vi "Camera Params OFF_Luan2024.05.01.vi"(8 "error in (no error)":errorcluster, 11 "IMAQDx session In":T1) -> (0 "error out":errorcluster, 3 "IMAQDx session out":T1)   [LabVIEW 2023]
uses:
  <vilib>/userDefined/High Color/IMAQdx.ctl
  <resource>/objmgr/imaqdx.rc
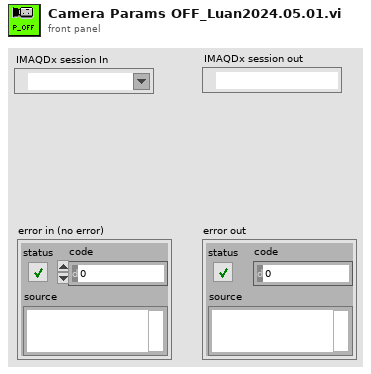
[diagram p1: front panel]
types:
  T1 = typedef "IMAQdx.ctl" = refnum<k21>
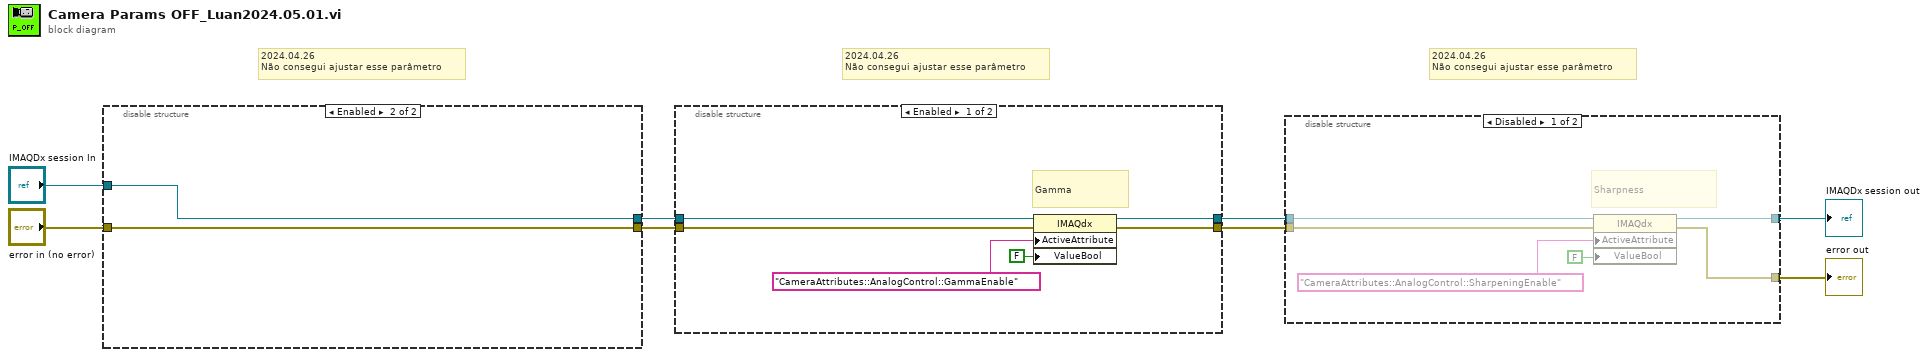
[diagram p0: block diagram]
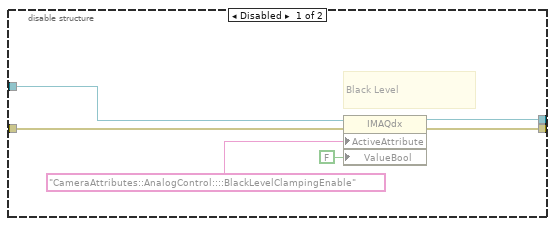
[diagram p4: hidden frame]
diagram:
  # "2024.04.26\nNão consegui ajustar esse parâmetro"
  # "2024.04.26\nNão consegui ajustar esse parâmetro"
  # "2024.04.26\nNão consegui ajustar esse parâmetro"
  n1 = disable-structure shown="Enabled" {
    disable-tunnel: [w14 w15] -> w6
    disable-tunnel: [w13 w16] -> w5
    disable-tunnel: "IMAQDx session In" -> [w11 w16]
    disable-tunnel: "error in (no error)" -> [w10 w15]
    frame Disabled {
      # "Black Level"
      n2 = property class="IMAQdx"(reference=w11, error in=w10, "ActiveAttribute"="CameraAttributes::AnalogControl::::BlackLevelClampingEnable", "ValueBool"=FALSE) -> (reference out=w13:T1, error out=w14:errorcluster)
    }
    frame Enabled {
    }
  }
  n3 = disable-structure shown="Enabled" {
    disable-tunnel: [w22 w23] -> w8
    disable-tunnel: [w21 w24] -> w7
    disable-tunnel: w6 -> [w20 w23]
    disable-tunnel: w5 -> [w19 w24]
    frame Enabled {
      # "Gamma"
      n4 = property class="IMAQdx"(reference=w19, error in=w20, "ActiveAttribute"="CameraAttributes::AnalogControl::GammaEnable", "ValueBool"=FALSE) -> (reference out=w21:T1, error out=w22:errorcluster)
    }
    frame Disabled {
    }
  }
  n5 = disable-structure shown="Disabled" {
    disable-tunnel: w8 -> [w30 w31]
    disable-tunnel: w7 -> [w29 w32]
    disable-tunnel: [w26 w32] -> w3
    disable-tunnel: [w25 w31] -> w2
    frame Disabled {
      # "Sharpness"
      n6 = property class="IMAQdx"(reference=w29, error in=w30, "ActiveAttribute"="CameraAttributes::AnalogControl::SharpeningEnable", "ValueBool"=FALSE) -> (reference out=w26:T1, error out=w25:errorcluster)
    }
    frame Enabled {
    }
  }
  "IMAQDx session out" <- w3
  "error out" <- w2
